vi "Spectral Analysis ME45 (2).vi"() -> ()   [LabVIEW 2022 SP3]
uses:
  <vilib>/express/express analysis/Spectral/Block/exnSpectralBlock spectral measurements peak poly.vi
  <vilib>/express/express analysis/Spectral/Block/exnSpectralBlock spectral measurements peak DDT.vi
  <vilib>/express/express analysis/Spectral/XNode/ExpressSpectralMeasurementsBlockNode.xnode
panel:
  in  "Controls":enum32{"Spectrum Analyzer"}(tab)
  in  "?":bool
  in  "?":bool
  in  "?":bool
  in  "Playback Sound":bool
  in  "Recording Duration (s)":dbl=5.0 caption="Duration (s)"
  in  "Sampling Rate (Hz)":dbl(slide) scale=0.0..44100.0
  in  "Recording Method":bool
  out "FFT":dynamicdata(graph)
  out "Raw Sound Data":dynamicdata(graph)
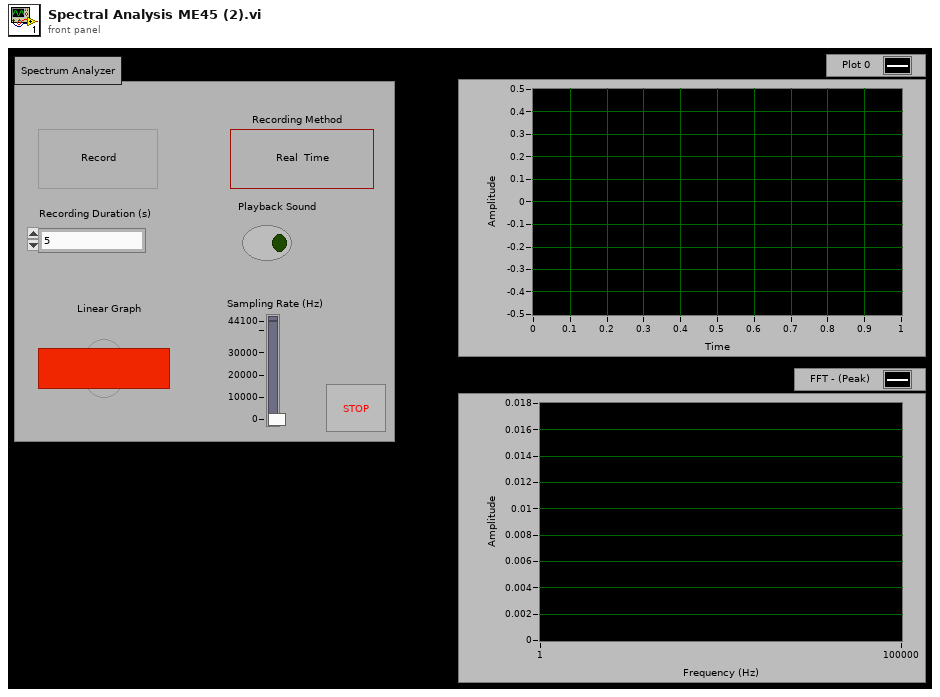
[diagram p1: front panel]
types:
  T1 = cluster{"averaging mode":u16, "weighting mode":u16, "number of averages":u32}
  T2 = cluster{"dB On (F)":bool, "unwrap phase (F)":bool, "convert to degree (F)":bool}
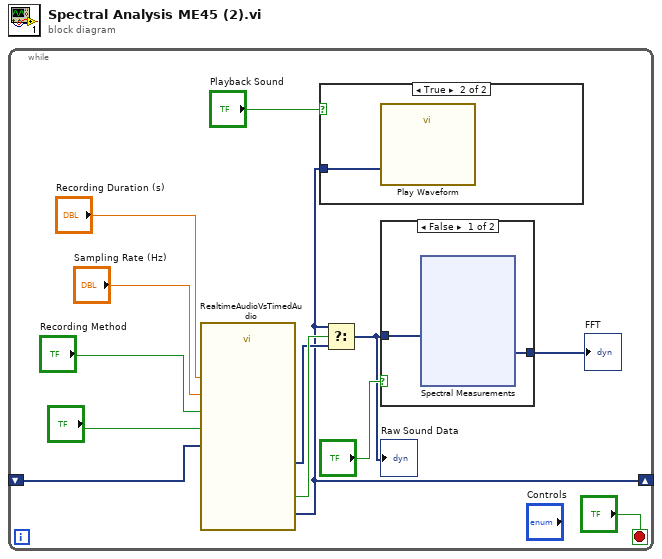
[diagram p0: block diagram]
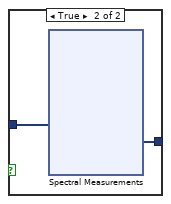
[diagram p2: hidden frame]
diagram:
  n1 = while {
    shift-right: [w4] -> _
    shift-left: _ -> [w5]
    stop <- "?" stop-if-true
    n2 = call "RealtimeAudioVsTimedAudio.vi"("Recording Duration (s)"="Recording Duration (s)", "Sample Rate (Hz)"="Sampling Rate (Hz)", "Waveform Buffer In"=w5, "Record Sound"="?", "FreeRecord or TimedRecord"="Recording Method") -> ("FreeRecord Out"=w7:dynamicdata, "RecordingType Status"=w8:bool, "Waveform Buffer Storage"=w4:dynamicdata)  [unwired: 3 in, 1 out]
    n3 = case shown="True" "Playback Sound" {
      tunnel: w4 -> [_ w38]
      frame False {
      }
      frame True {
        n4 = call "Play Waveform"("Data"=w38) -> ()  [unwired: 18 in, 1 out]
      }
    }
    n5 = Select(t=w4, s=w8, f=w7) -> (s? t:f=w6:dynamicdata)
    "Raw Sound Data" <- w6
    n6 = case shown="False" "?" {
      tunnel: [w15 w27] -> w12
      tunnel: w6 -> [w14 w26]
      frame False {
        n7 = xnode "Spectral Measurements"("Signals"=w14) -> ("FFT - (Peak)"=w15:dynamicdata)  [unwired: 1 in, 2 out]
      }
      frame True {
        n8 = xnode "Spectral Measurements"("Signals"=w26) -> ("FFT - (Peak)"=w27:dynamicdata)  [unwired: 1 in, 2 out]
      }
    }
    "FFT" <- w12
  }
